vi "Obtain Message Queue.vi"(8 "error in (no error)":errorcluster) -> (0 "error out":errorcluster, 3 "Message Queue":refnum<queue>)   [LabVIEW 2021, in "RMU Message Queue.lvlib"]
doc: "Create a queue with the Message Cluster data type."
uses:
  RMU Message Queue.lvlib
  Message Cluster.ctl
  controls/developer_test sequence.ctl
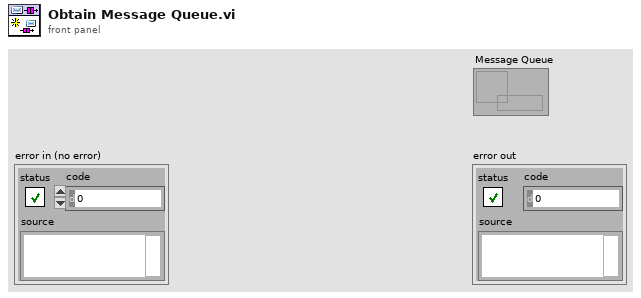
[diagram p1: front panel]
types:
  T1 = typedef "RMU Message Queue.lvlib/Message Cluster.ctl" = cluster{"test sequence":T2, "Message Data":variant}
  T2 = typedef "developer_test sequence.ctl" = enum16{"Update Display", "User Login", "Initialise", "Init Devices", "Idle State", "test steup", "Abort", "Start Display Board Auto Testing", "Scan Barcode", "Checking TEMP at Thermistor 1", "Checking TEMP at Thermistor 2", "Checking TEMP at Thermistor 3", "Checking TEMP at Thermistor 4 (Ambient)", "Voltage Health Check", "INSULATION Resistance test (Baseplate to Negative)", "INSULATION Resistance test (Baseplate to Positive)", "WELD Resistance Test", "Stop Display Board Auto Testing", "All Pass", "Fail", "Report", "Error", "Confirm Quit", "Exit"}
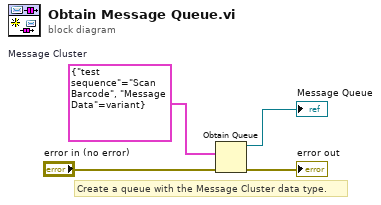
[diagram p0: block diagram]
diagram:
  w4 = T1 {"test sequence"=enum."Scan Barcode", "Message Data"=variant}  # Message Cluster
  # "Create a queue with the Message Cluster data type."
  n1 = Obtain Queue(element data type=w4, error in (no error)="error in (no error)") -> (queue out=→"Message Queue":refnum<queue>, error out=→"error out":errorcluster)  [unwired: 3 in, 1 out]
